vi "BCM_CmdStr_284.vi"(1 "BCM命令输入":T1 {"BCM电源模式" items=["关闭", "ACC", "开启", "预留", "START"]; "设防提示类型设置" items=["无", "亮灯并鸣笛", "亮灯", "鸣笛"]; "RLS下雨关窗模式" items=["关", "开", "预留", "错误"]; "防盗报警状态" items=["报警", "预报警", "禁止报警", "提醒", "警报", "部分报警", "未用"]; "自动开关窗设置" items=["禁止", "RKE长按控制", "车钥匙控制", "预留"]; "伴我回家时间选择" items=["无", "30s", "60s", "90s"]; "BCM提示引擎盖开关" items=["关闭", "半开", "预留", "无效"]; "后车窗加热器激活" items=["未激活", "激活", "预留", "无效"]}) -> (0 "CmdStr":string)   [LabVIEW 2013]
uses:
  BCM_284.ctl
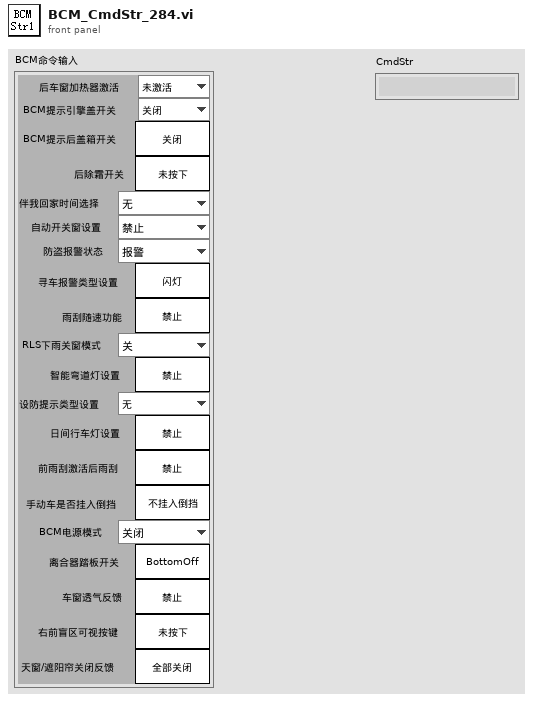
[diagram p1: front panel]
types:
  T1 = typedef "BCM_284.ctl" = cluster{"后车窗加热器激活":u16, "BCM提示引擎盖开关":u16, "BCM提示后盖箱开关":bool, "后除霜开关":bool, "伴我回家时间选择":u16, "自动开关窗设置":u16, "防盗报警状态":u16, "寻车报警类型设置":bool, "雨刮随速功能":bool, "RLS下雨关窗模式":u16, "智能弯道灯设置":bool, "设防提示类型设置":u16, "日间行车灯设置":bool, "前雨刮激活后雨刮":bool, "手动车是否挂入倒挡":bool, "BCM电源模式":u16, "离合器踏板开关":bool, "车窗透气反馈":bool, "右前盲区可视按键":bool, "天窗/遮阳帘关闭反馈":bool}
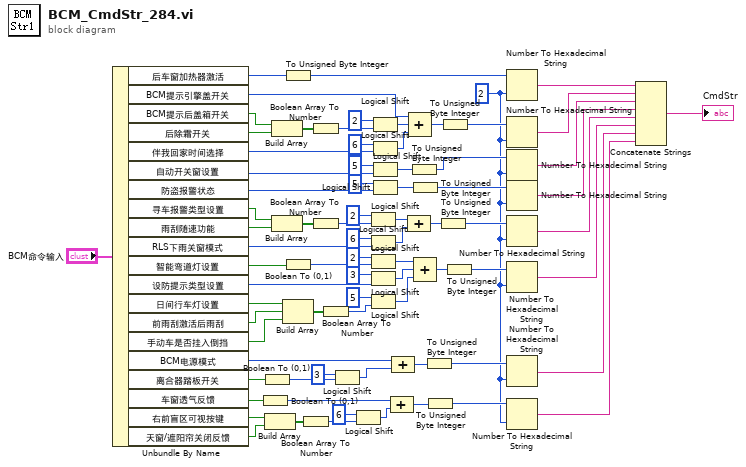
[diagram p0: block diagram]
diagram:
  w2 = 2
  n1 = Unbundle By Name("BCM命令输入") -> ("后车窗加热器激活"=w76:u16, "BCM提示引擎盖开关"=w68:u16, "BCM提示后盖箱开关"=w75:bool, "后除霜开关"=w74:bool, "伴我回家时间选择"=w65:u16, "自动开关窗设置"=w63:u16, "防盗报警状态"=w60:u16, "寻车报警类型设置"=w57:bool, "雨刮随速功能"=w56:bool, "RLS下雨关窗模式"=w50:u16, "智能弯道灯设置"=w47:bool, "设防提示类型设置"=w45:u16, "日间行车灯设置"=w41:bool, "前雨刮激活后雨刮"=w40:bool, "手动车是否挂入倒挡"=w39:bool, "BCM电源模式"=w32:u16, "离合器踏板开关"=w33:bool, "车窗透气反馈"=w27:bool, "右前盲区可视按键"=w24:bool, "天窗/遮阳帘关闭反馈"=w25:bool)
  n2 = Boolean To (0,1)(Boolean=w27) -> (0, 1=w26:i16)
  n3 = Boolean To (0,1)(Boolean=w33) -> (0, 1=w30:i16)
  n4 = Build Array(w24, w25) -> (w21:bool[])
  n5 = Build Array(w75, w74) -> (w72:bool[])
  n6 = Build Array(w57, w56) -> (w58:bool[])
  n7 = To Unsigned Byte Integer(number=w76) -> (unsigned 8bit integer=w4:u8)
  n8 = Boolean To (0,1)(Boolean=w47) -> (0, 1=w46:i16)
  n9 = Build Array(w41, w40, w39) -> (w38:bool[])
  n10 = Boolean Array To Number(Boolean array=w21) -> (number=w20:u32)
  n11 = Boolean Array To Number(Boolean array=w72) -> (number=w70:u32)
  n12 = Boolean Array To Number(Boolean array=w58) -> (number=w54:u32)
  n13 = Boolean Array To Number(Boolean array=w38) -> (number=w36:u32)
  n14 = Logical Shift(y=u8 3, x=w30) -> (x << y=w29:i16)
  n15 = Logical Shift(y=u8 6, x=w20) -> (x << y=w22:u32)
  n16 = Logical Shift(y=u8 2, x=w54) -> (x << y=w53:u32)
  n17 = Logical Shift(y=u8 6, x=w50) -> (x << y=w51:u16)
  n18 = Logical Shift(y=u8 2, x=w46) -> (x << y=w43:i16)
  n19 = Logical Shift(y=u8 3, x=w45) -> (x << y=w42:u16)
  n20 = Logical Shift(y=u8 5, x=w36) -> (x << y=w35:u32)
  n21 = Logical Shift(y=u8 2, x=w70) -> (x << y=w69:u32)
  n22 = Logical Shift(y=u8 6, x=w65) -> (x << y=w66:u16)
  n23 = Logical Shift(y=u8 5, x=w63) -> (x << y=w62:u16)
  n24 = Logical Shift(y=u8 5, x=w60) -> (x << y=w59:u16)
  n25 = Compound Arithmetic op=ADD(w26, w22) -> (w19:u32)
  n26 = Compound Arithmetic op=ADD(w32, w29) -> (w28:u16)
  n27 = Compound Arithmetic op=ADD(w53, w51) -> (w49:u32)
  n28 = Compound Arithmetic op=ADD(w68, w69, w66) -> (w73:u32)
  n29 = To Unsigned Byte Integer(number=w62) -> (unsigned 8bit integer=w16:u8)
  n30 = To Unsigned Byte Integer(number=w59) -> (unsigned 8bit integer=w14:u8)
  n31 = Compound Arithmetic op=ADD(w43, w42, w35) -> (w34:u32)
  n32 = To Unsigned Byte Integer(number=w28) -> (unsigned 8bit integer=w8:u8)
  n33 = To Unsigned Byte Integer(number=w19) -> (unsigned 8bit integer=w6:u8)
  n34 = To Unsigned Byte Integer(number=w49) -> (unsigned 8bit integer=w12:u8)
  n35 = To Unsigned Byte Integer(number=w73) -> (unsigned 8bit integer=w18:u8)
  n36 = To Unsigned Byte Integer(number=w34) -> (unsigned 8bit integer=w10:u8)
  n37 = Number To Hexadecimal String(1:w2, 2:w4) -> (0:w3:string)
  n38 = Number To Hexadecimal String(1:w2, 2:w18) -> (0:w17:string)
  n39 = Number To Hexadecimal String(1:w2, 2:w16) -> (0:w15:string)
  n40 = Number To Hexadecimal String(1:w2, 2:w14) -> (0:w13:string)
  n41 = Number To Hexadecimal String(1:w2, 2:w12) -> (0:w11:string)
  n42 = Number To Hexadecimal String(1:w2, 2:w10) -> (0:w9:string)
  n43 = Number To Hexadecimal String(1:w2, 2:w8) -> (0:w7:string)
  n44 = Number To Hexadecimal String(1:w2, 2:w6) -> (0:w5:string)
  n45 = Concatenate Strings(w3, w17, w15, w13, w11, w9, w7, w5) -> (→"CmdStr":string)
